vi "fgv_stop.vi"(7 "cmd":enum16{"default", "ini", "stop"}(ring), 8 "error in":errorcluster) -> (0 "error out":errorcluster, 3 "stop":bool)   [LabVIEW 2017]
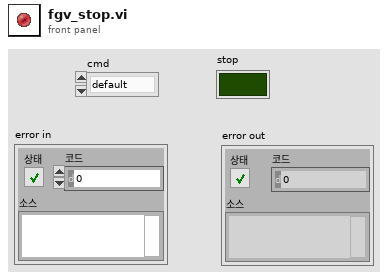
[diagram p1: front panel]
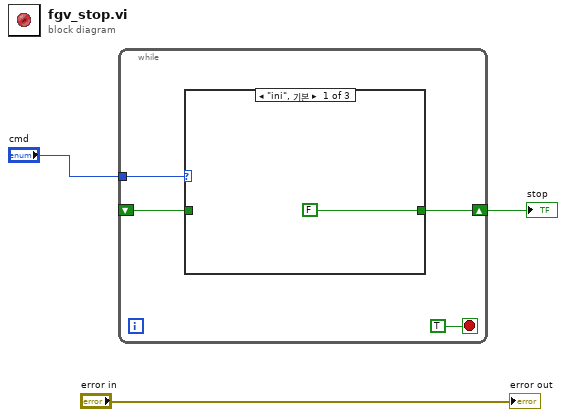
[diagram p0: block diagram]
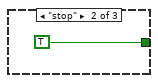
[diagram p2: hidden frame]
diagram:
  n1 = while {
    tunnel: "cmd" -> [w7]
    shift-right: [w5] -> w2
    shift-left: _ -> [w4]
    stop <- TRUE stop-if-true
    n2 = case shown="\"ini\", 기본" w7 {
      tunnel: [FALSE TRUE w10] -> w5
      tunnel: w4 -> [_ _ w10]
      frame "ini", Default {
      }
      frame "stop" {
      }
      frame "default" {
      }
    }
  }
  "stop" <- w2
  "error out" <- "error in"
